vi "Analog Init.vi"(8 "error in (no error)":errorcluster) -> (0 "error out":errorcluster, 3 "Analog":T1)   [LabVIEW 2020]
uses:
  <vilib>/High Genius/HG_WSI_Tookit/Dependencies/Library/Analog In/Analog In.lvclass
  C:/Program Files (x86)/National Instruments/LabVIEW 2020/vi.lib/High Genius/HG_WSI_Tookit/Dependencies/Library/HG_LIB/HG_LIB.lvclass
  <vilib>/High Genius/HG_WSI_Tookit/Dependencies/Library/HG_LIB/HG_LIB.lvclass
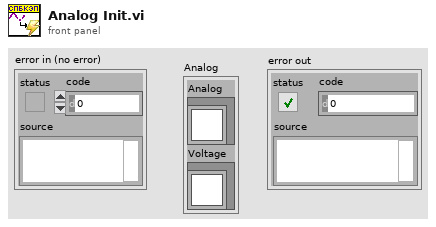
[diagram p1: front panel]
types:
  T1 = cluster{"Analog":refnum<class "Analog In.lvclass">, "Voltage":refnum<class "Analog In.lvclass">}
  T2 = enum16{"DI", "DO", "AI", "Pulse", "PWM", "ISQ", "ENC", "CAN", "IIC", "IMU"}
  T3 = enum16{"0", "1", "2", "3", "4", "5", "6", "7", "8", "9", "10", "11", "12", "13", "14", "15", "16", "17", "18", "19", "20", "21", "22", "23", "24", "25"}
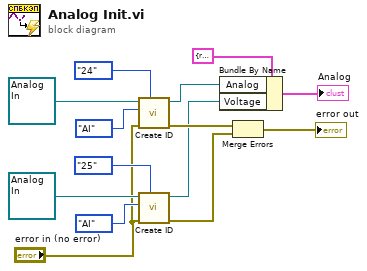
[diagram p0: block diagram]
diagram:
  n1 = call <vilib>:"Create ID.vi"("NO"=T3."24", "error in (no error)"="error in (no error)", "Function"=T2."AI", "HG_LIB in"=refnum<class "Analog In.lvclass"> refnum ("Analog In.lvclass")) -> ("error out"=w8:errorcluster, "HG_LIB out"=w2:refnum<class "Analog In.lvclass">)  [unwired: 6 in]
  n2 = call <vilib>:"Create ID.vi"("NO"=T3."25", "error in (no error)"="error in (no error)", "Function"=T2."AI", "HG_LIB in"=refnum<class "Analog In.lvclass"> refnum ("Analog In.lvclass")) -> ("error out"=w9:errorcluster, "HG_LIB out"=w1:refnum<class "Analog In.lvclass">)  [unwired: 6 in]
  n3 = Bundle By Name(cluster=T1 {"Analog"=refnum, "Voltage"=refnum} ("HG_LIB out"), "Analog"=w2, "Voltage"=w1) -> (→"Analog":T1)
  n4 = Merge Errors(w8, w9) -> (→"error out":errorcluster)
